vi "GetDataSetValuesFromDVR.vi"(7 "delete dvr":bool, 8 "error in (no error)":errorcluster, 11 "values dvr":refnum<data-value>) -> (0 "error out":errorcluster, 3 "values":sgl[](array[numeric]))   [LabVIEW 2017, in "DataEventCreator.lvlib"]
uses:
  <vilib>/addons/InsightCM/Devices/Shared/Common/DataEventCreator/DataEventCreator.lvlib
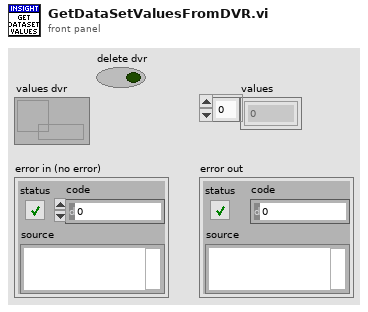
[diagram p1: front panel]
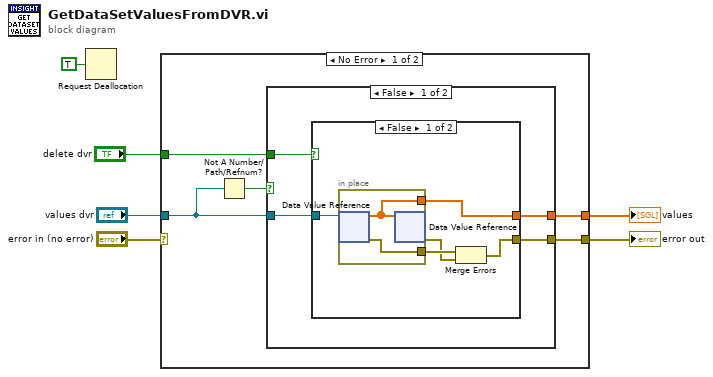
[diagram p0: block diagram]
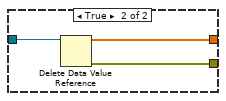
[diagram p2: hidden frame]
diagram:
  n1 = Request Deallocation(TRUE ("flag")) -> ()
  n2 = case shown="No Error" "error in (no error)" {
    selector: "error in (no error)" -> [_ w26]
    tunnel: [w7 w26] -> w6
    tunnel: [w11 _] -> w5
    tunnel: "values dvr" -> [w9 _]
    tunnel: "delete dvr" -> [w8 _]
    frame No Error {
      n3 = Not A Number/Path/Refnum?(number/path/refnum=w9) -> (NaN/Path/Refnum?=w10:bool)
      n4 = case shown="False" w10 {
        tunnel: [w15 _] -> w11
        tunnel: w9 -> [w14 _]
        tunnel: w8 -> [w13 _]
        tunnel: [w12 _] -> w7
        frame False {
          n5 = case shown="False" w13 {
            tunnel: [w19 w25] -> w12
            tunnel: [w16 w24] -> w15
            tunnel: w14 -> [w20 w23]
            frame False {
              n6 = in-place {
                in-place-border: [w22] -> w18
                in-place-border: [w21] -> w16
                n7 = in-place-dvr #1(w20) -> (w21:sgl[], w22:errorcluster)
                n8 = in-place-dvr #1(w21) -> (w17:errorcluster)  [unwired: 1 out]
              }
              n9 = Merge Errors(w18, w17) -> (w19:errorcluster)
            }
            frame True {
              n10 = Delete Data Value Reference(data value reference=w23) -> (data value=w24:sgl[], error out=w25:errorcluster)  [unwired: 1 in]
            }
          }
        }
        frame True {
        }
      }
    }
    frame Error {
    }
  }
  "error out" <- w6
  "values" <- w5
